vi "Build Edge Graph Legend.vi"() -> (3 "Edge Legend Graph":string)   [LabVIEW 2021, in "TAF Proj Document Type.lvlib" / "TAF Proj.lvclass"]
uses:
  <vilib>/Wovalab/AntiDoc/Document Type/Add-ons/LabVIEW TAF Project/TAF Proj/TAF Proj.lvclass
  <vilib>/Wovalab/AntiDoc/GraphBuilder/Renderer/Graphviz/Graphviz.lvclass
  C:/Program Files (x86)/National Instruments/LabVIEW 2021/vi.lib/Wovalab/AntiDoc/GraphBuilder/Renderer/Renderer.lvclass
  <vilib>/Wovalab/AntiDoc/GraphBuilder/Graph/Graph.lvclass
  <vilib>/Wovalab/AntiDoc/GraphBuilder/Shapes/Edge/Graphviz/Graphviz Edge Shape.lvclass
  <vilib>/Wovalab/AntiDoc/GraphBuilder/Shapes/Node/Graphviz/Graphviz Node Shape.lvclass
  <vilib>/Wovalab/AntiDoc/GraphBuilder/Shapes/Edge/Graphviz/Shape.ctl
  <vilib>/Wovalab/AntiDoc/GraphBuilder/Shapes/Edge/Graphviz/Colors.ctl
  <vilib>/Wovalab/AntiDoc/GraphBuilder/Shapes/Node/Graphviz/Colors.ctl
  <vilib>/Wovalab/AntiDoc/GraphBuilder/Shapes/Node/Graphviz/Shape.ctl
  <vilib>/Wovalab/AntiDoc/GraphBuilder/Renderer/Graphviz/Graph Direction.ctl
  <vilib>/Wovalab/AntiDoc/GraphBuilder/Edge/Edge.lvclass
  <vilib>/Wovalab/AntiDoc/GraphBuilder/Renderer/Graphviz/Specific Edge Shape Def.ctl
  <vilib>/Wovalab/AntiDoc/GraphBuilder/Node/Node.lvclass
  <vilib>/Wovalab/AntiDoc/GraphBuilder/Renderer/Graphviz/Specific Node Shape Def.ctl
  <vilib>/Wovalab/AntiDoc/Document Type/Add-ons/LabVIEW TAF Project/TAF Proj Document Type.lvlib
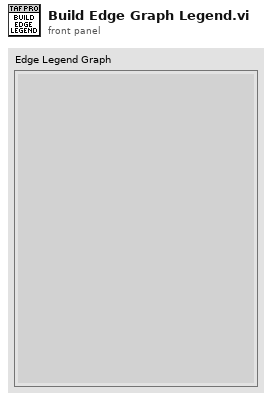
[diagram p1: front panel]
types:
  T1 = typedef "GraphBuilder.lvlib/Graphviz Edge Shape.lvclass/Shape.ctl" = enum16{"box", "lbox", "rbox", "obox", "olbox", "orbox", "crow", "lcrow", "rcrow", "diamond", "ldiamond", "rdiamond", "odiamond", "oldiamond", "ordiamond", "dot", "odot", "inv", "linv", "rinv", "oinv", "olinv", "orinv", "none", "normal", "lnormal", "rnormal", "onormal", "olnormal", "ornormal", "tee", "ltee", "rtee", "vee", "lvee", "rvee", "curve", "lcurve", "rcurve", "icurve", "licurve", "ricurve"}
  T2 = typedef "GraphBuilder.lvlib/Graphviz.lvclass/Specific Edge Shape Def.ctl" = cluster{"Source Node ID":string, "Target Node ID":string, "Caption":string, "Graphviz Edge Shape":refnum<class "Graphviz Edge Shape.lvclass">}
  T3 = typedef "GraphBuilder.lvlib/Graphviz.lvclass/Graph Direction.ctl" = enum16{"Top to Bottom", "Left To Right", "Bottom to Top", "Right to Left"}
  T4 = typedef "GraphBuilder.lvlib/Graphviz Node Shape.lvclass/Shape.ctl" = enum16{"box", "polygon", "ellipse", "oval", "circle", "point", "egg", "triangle", "plaintext", "plain", "diamond", "trapezium", "parallelogram", "house", "pentagon", "hexagon", "septagon", "octagon", "doublecircle", "doubleoctagon", "tripleoctagon", "invtriangle", "invtrapezium", "invhouse", "Mdiamond", "Msquare", "Mcircle", "rect", "rectangle", "square", "star", "none", "underline", "cylinder", "note", "tab", "folder", "box3D", "component", "promoter", "cds", "terminator", "utr", "primersite", "restrictionsite", "fivepoverhang", "threepoverhang", "noverhang", "assembly", "signature", "insulator", "ribosite", "rnastab", "proteasesite", "proteinstab", "rpromoter", "rarrow", "larrow", "lpromoter"}
  T5 = typedef "GraphBuilder.lvlib/Graphviz Node Shape.lvclass/Colors.ctl" = enum16{"aliceblue", "antiquewhite", "aqua", "aquamarine", "azure", "beige", "bisque", "black", "blanchedalmond", "blue", "blueviolet", "brown", "burlywood", "cadetblue", "chartreuse", "chocolate", "coral", "cornflowerblue", "cornsilk", "crimson", "cyan", "darkblue", "darkcyan", "darkgoldenrod", "darkgray", "darkgreen", "darkgrey", "darkkhaki", "darkmagenta", "darkolivegreen", "darkorange", "darkorchid", "darkred", "darksalmon", "darkseagreen", "darkslateblue", "darkslategray", "darkslategrey", "darkturquoise", "darkviolet", "deeppink", "deepskyblue", "dimgray", "dimgrey", "dodgerblue", "firebrick", "floralwhite", "forestgreen", "fuchsia", "gainsboro", "ghostwhite", "gold", "goldenrod", "gray", "green", "greenyellow", "grey", "honeydew", "hotpink", "indianred", "indigo", "ivory", "khaki", "lavender", "lavenderblush", "lawngreen", "lemonchiffon", "lightblue", "lightcoral", "lightcyan", "lightgoldenrodyellow", "lightgray", "lightgreen", "lightgrey", "lightpink", "lightsalmon", "lightseagreen", "lightskyblue", "lightslategray", "lightslategrey", "lightsteelblue", "lightyellow", "lime", "limegreen", "linen", "magenta", "maroon", "mediumaquamarine", "mediumblue", "mediumorchid", "mediumpurple", "mediumseagreen", "mediumslateblue", "mediumspringgreen", "mediumturquoise", "mediumvioletred", "midnightblue", "mintcream", "mistyrose", "moccasin", "navajowhite", "navy", "oldlace", "olive", "olivedrab", "orange", "orangered", "orchid", "palegoldenrod", "palegreen", "paleturquoise", "palevioletred", "papayawhip", "peachpuff", "peru", "pink", "plum", "powderblue", "purple", "red", "rosybrown", "royalblue", "saddlebrown", "salmon", "sandybrown", "seagreen", "seashell", "sienna", "silver", "skyblue", "slateblue", "slategray", "slategrey", "snow", "springgreen", "steelblue", "tan", "teal", "thistle", "tomato", "turquoise", "violet", "wheat", "white", "whitesmoke", "yellow", "yellowgreen"}
  T6 = typedef "GraphBuilder.lvlib/Graphviz Edge Shape.lvclass/Colors.ctl" = enum16{"aliceblue", "antiquewhite", "aqua", "aquamarine", "azure", "beige", "bisque", "black", "blanchedalmond", "blue", "blueviolet", "brown", "burlywood", "cadetblue", "chartreuse", "chocolate", "coral", "cornflowerblue", "cornsilk", "crimson", "cyan", "darkblue", "darkcyan", "darkgoldenrod", "darkgray", "darkgreen", "darkgrey", "darkkhaki", "darkmagenta", "darkolivegreen", "darkorange", "darkorchid", "darkred", "darksalmon", "darkseagreen", "darkslateblue", "darkslategray", "darkslategrey", "darkturquoise", "darkviolet", "deeppink", "deepskyblue", "dimgray", "dimgrey", "dodgerblue", "firebrick", "floralwhite", "forestgreen", "fuchsia", "gainsboro", "ghostwhite", "gold", "goldenrod", "gray", "green", "greenyellow", "grey", "honeydew", "hotpink", "indianred", "indigo", "ivory", "khaki", "lavender", "lavenderblush", "lawngreen", "lemonchiffon", "lightblue", "lightcoral", "lightcyan", "lightgoldenrodyellow", "lightgray", "lightgreen", "lightgrey", "lightpink", "lightsalmon", "lightseagreen", "lightskyblue", "lightslategray", "lightslategrey", "lightsteelblue", "lightyellow", "lime", "limegreen", "linen", "magenta", "maroon", "mediumaquamarine", "mediumblue", "mediumorchid", "mediumpurple", "mediumseagreen", "mediumslateblue", "mediumspringgreen", "mediumturquoise", "mediumvioletred", "midnightblue", "mintcream", "mistyrose", "moccasin", "navajowhite", "navy", "oldlace", "olive", "olivedrab", "orange", "orangered", "orchid", "palegoldenrod", "palegreen", "paleturquoise", "palevioletred", "papayawhip", "peachpuff", "peru", "pink", "plum", "powderblue", "purple", "red", "rosybrown", "royalblue", "saddlebrown", "salmon", "sandybrown", "seagreen", "seashell", "sienna", "silver", "skyblue", "slateblue", "slategray", "slategrey", "snow", "springgreen", "steelblue", "tan", "teal", "thistle", "tomato", "turquoise", "violet", "wheat", "white", "whitesmoke", "yellow", "yellowgreen"}
  T7 = typedef "GraphBuilder.lvlib/Graphviz.lvclass/Specific Node Shape Def.ctl" = cluster{"Node ID":string, "Graphviz Node Shape":refnum<class "Graphviz Node Shape.lvclass">}
  T8 = typedef "GraphBuilder.lvlib/Graphviz Edge Shape.lvclass/Style.ctl" = enum8{"filled", "invisible", "diagonals", "rounded", "dashed", "dotted", "solid", "bold"}
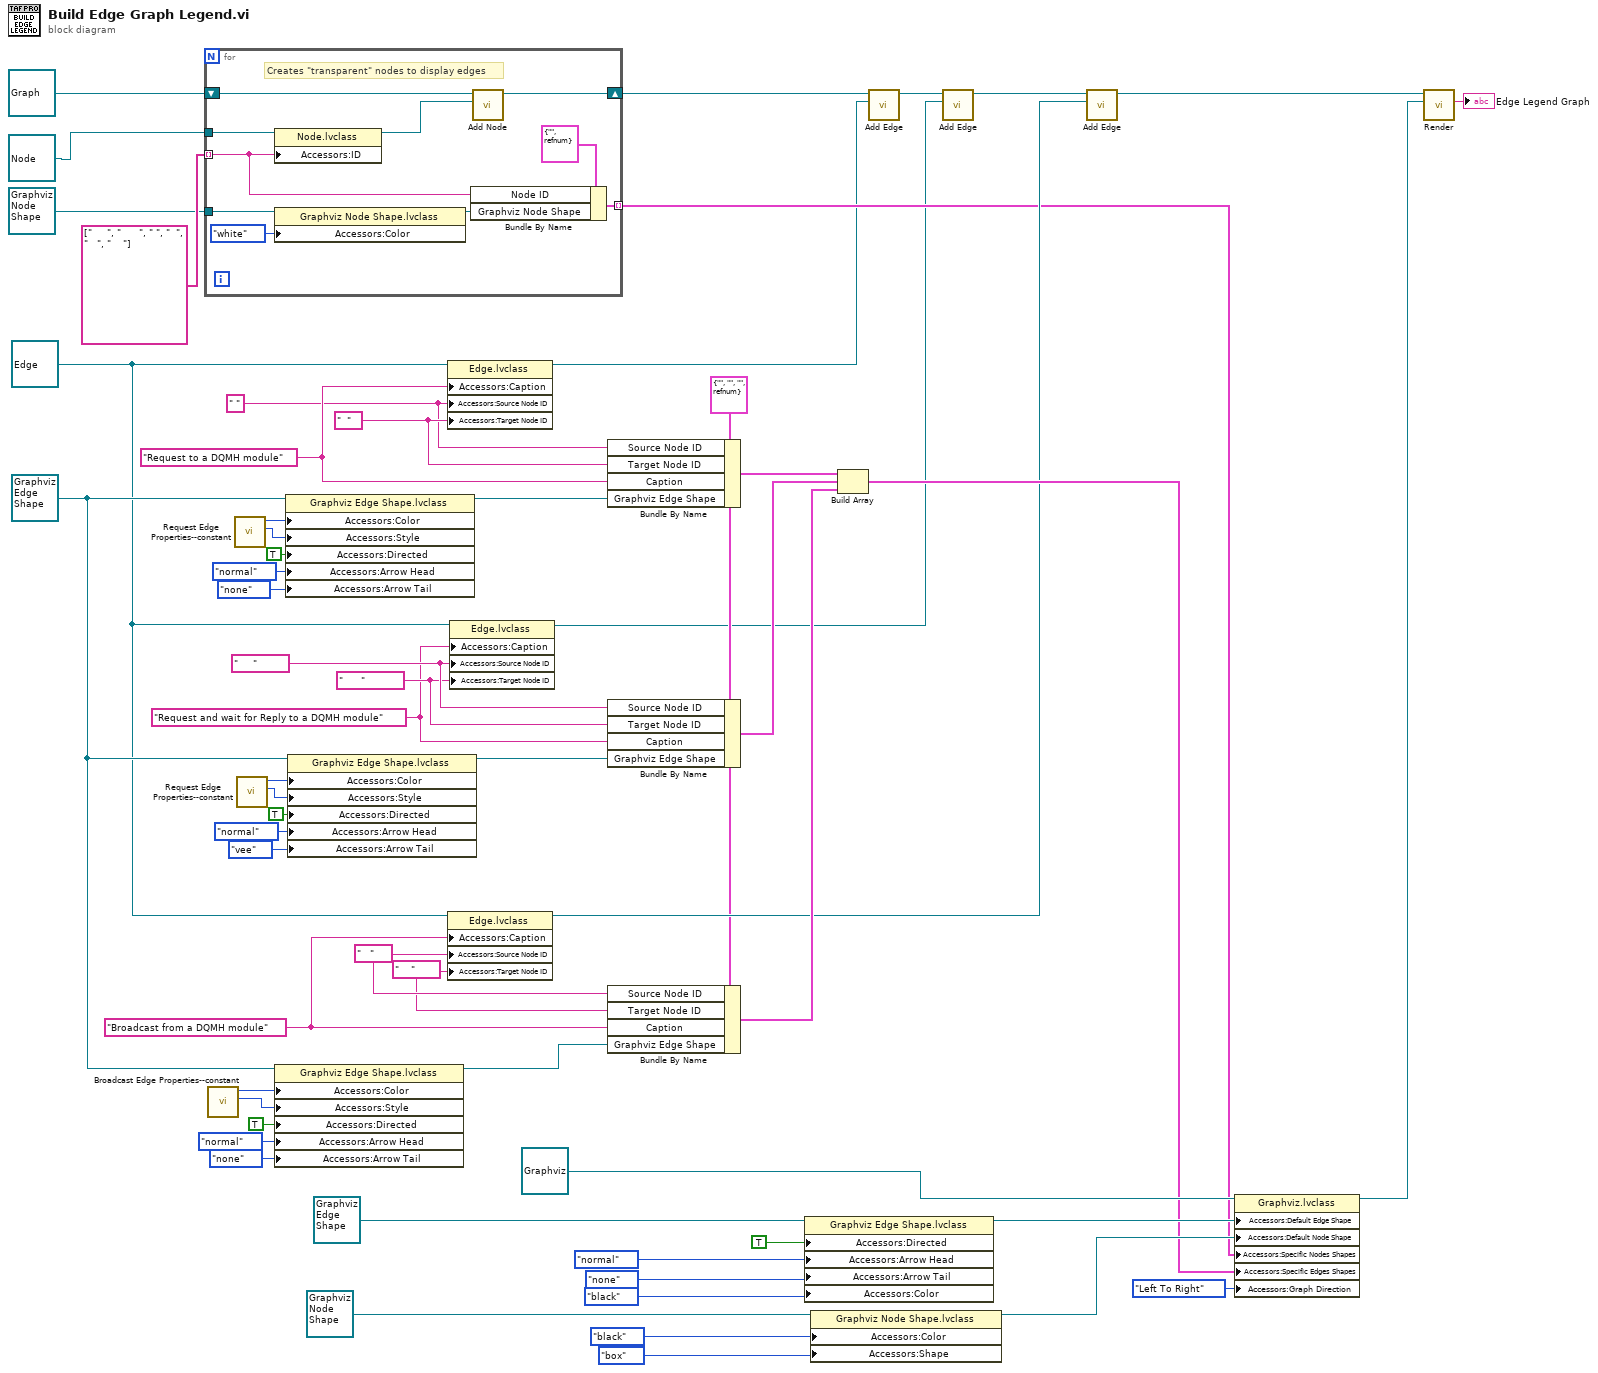
[diagram p0: block diagram]
diagram:
  w14 = "     "
  w13 = "      "
  w12 = "Request and wait for Reply to a DQMH module" ("Caption")
  w22 = " "
  w26 = "    "
  w27 = "   "
  w28 = "  "
  w38 = "Broadcast from a DQMH module" ("Caption")
  w5 = refnum<class "Graphviz Edge Shape.lvclass"> refnum ("Graphviz Edge Shape")
  w7 = T2 {"Source Node ID"="", "Target Node ID"="", "Caption"="", "Graphviz Edge Shape"=refnum} ("Specific Edge Shape")
  w32 = "Request to a DQMH module" ("Caption")
  w4 = refnum<class "Edge.lvclass"> refnum ("Edge")
  n1 = for {
    tunnel: string[] ["     ", "      ", " ", "  ", "   ", "    "] -> [w70] mode=indexing
    tunnel: [w66] -> w29 mode=indexing
    tunnel: refnum<class "Graphviz Node Shape.lvclass"> refnum ("GraphBuilder.lvlib:Graphviz Node Shape.lvclass") -> [w65]
    tunnel: refnum<class "Node.lvclass"> refnum ("GraphBuilder.lvlib:Node.lvclass") -> [w64]
    shift-right: [w62] -> w19
    shift-left: refnum<class "Graph.lvclass"> refnum ("GraphBuilder.lvlib:Graph.lvclass") -> [w63]
    # "Creates \"transparent\" nodes to display edges"
    n2 = property class="Node.lvclass"(reference=w64, "Accessors:ID"=w70) -> (reference out=w61:refnum<class "Node.lvclass">)  [unwired: 1 in, 1 out]
    n3 = property class="Graphviz Node Shape.lvclass"(reference=w65, "Accessors:Color"=Colors."white" ("Color")) -> (reference out=w69:refnum<class "Graphviz Node Shape.lvclass">)  [unwired: 1 in, 1 out]
    n4 = Bundle By Name(cluster=T7 {"Node ID"="", "Graphviz Node Shape"=refnum} ("Specific Node Shape"), "Node ID"=w70, "Graphviz Node Shape"=w69) -> (w66:T7)
    n5 = call-dynamic "Add Node.vi"("Node"=w61, "Graph in"=w63) -> ("Graph out"=w62:refnum<class "Graph.lvclass">)  [unwired: 8 in, 1 out]
  }
  n6 = call <vilib>:"Broadcast Edge Properties--constant.vi"() -> ("Style"=w35:T8, "Edge Color"=w36:T6)  [unwired: 10 in]
  n7 = call <vilib>:"Request Edge Properties--constant.vi"() -> ("Style"=w45:T8, "Edge Color"=w46:T6)  [unwired: 10 in]
  n8 = call <vilib>:"Request Edge Properties--constant.vi"() -> ("Style"=w10:T8, "Edge Color"=w9:T6)  [unwired: 10 in]
  n9 = property class="Graphviz Edge Shape.lvclass"(reference=w5, "Accessors:Color"=w36, "Accessors:Style"=w35, "Accessors:Directed"=TRUE ("Directed"), "Accessors:Arrow Head"=Shape."normal" ("Arrow Head"), "Accessors:Arrow Tail"=Shape."none" ("Arrow Tail")) -> (reference out=w39:refnum<class "Graphviz Edge Shape.lvclass">)  [unwired: 1 in, 1 out]
  n10 = property class="Graphviz Edge Shape.lvclass"(reference=w5, "Accessors:Color"=w46, "Accessors:Style"=w45, "Accessors:Directed"=TRUE ("Directed"), "Accessors:Arrow Head"=Shape."normal" ("Arrow Head"), "Accessors:Arrow Tail"=Shape."none" ("Arrow Tail")) -> (reference out=w47:refnum<class "Graphviz Edge Shape.lvclass">)  [unwired: 1 in, 1 out]
  n11 = property class="Graphviz Edge Shape.lvclass"(reference=w5, "Accessors:Color"=w9, "Accessors:Style"=w10, "Accessors:Directed"=TRUE ("Directed"), "Accessors:Arrow Head"=Shape."normal" ("Arrow Head"), "Accessors:Arrow Tail"=Shape."vee" ("Arrow Tail")) -> (reference out=w8:refnum<class "Graphviz Edge Shape.lvclass">)  [unwired: 1 in, 1 out]
  n12 = property class="Edge.lvclass"(reference=w4, "Accessors:Caption"=w32, "Accessors:Source Node ID"=w22, "Accessors:Target Node ID"=w28) -> (reference out=w23:refnum<class "Edge.lvclass">)  [unwired: 1 in, 1 out]
  n13 = property class="Edge.lvclass"(reference=w4, "Accessors:Caption"=w38, "Accessors:Source Node ID"=w27, "Accessors:Target Node ID"=w26) -> (reference out=w34:refnum<class "Edge.lvclass">)  [unwired: 1 in, 1 out]
  n14 = property class="Edge.lvclass"(reference=w4, "Accessors:Caption"=w12, "Accessors:Source Node ID"=w14, "Accessors:Target Node ID"=w13) -> (reference out=w1:refnum<class "Edge.lvclass">)  [unwired: 1 in, 1 out]
  n15 = Bundle By Name(cluster=w7, "Source Node ID"=w22, "Target Node ID"=w28, "Caption"=w32, "Graphviz Edge Shape"=w47) -> (w43:T2)
  n16 = Bundle By Name(cluster=w7, "Source Node ID"=w14, "Target Node ID"=w13, "Caption"=w12, "Graphviz Edge Shape"=w8) -> (w6:T2)
  n17 = Bundle By Name(cluster=w7, "Source Node ID"=w27, "Target Node ID"=w26, "Caption"=w38, "Graphviz Edge Shape"=w39) -> (w37:T2)
  n18 = property class="Graphviz Edge Shape.lvclass"(reference=refnum<class "Graphviz Edge Shape.lvclass"> refnum ("GraphBuilder.lvlib:Graphviz Edge Shape.lvclass"), "Accessors:Directed"=TRUE ("Directed"), "Accessors:Arrow Head"=Shape."normal" ("Arrow Head"), "Accessors:Arrow Tail"=Shape."none" ("Arrow Tail"), "Accessors:Color"=Colors."black" ("Color")) -> (reference out=w58:refnum<class "Graphviz Edge Shape.lvclass">)  [unwired: 1 in, 1 out]
  n19 = property class="Graphviz Node Shape.lvclass"(reference=refnum<class "Graphviz Node Shape.lvclass"> refnum ("GraphBuilder.lvlib:Graphviz Node Shape.lvclass"), "Accessors:Color"=Colors."black" ("Color"), "Accessors:Shape"=Shape."box" ("Shape")) -> (reference out=w59:refnum<class "Graphviz Node Shape.lvclass">)  [unwired: 1 in, 1 out]
  n20 = Build Array(w43, w6, w37) -> (w42:T2[])
  n21 = call-dynamic "Add Edge.vi"("Edge"=w23, "Graph in"=w19) -> ("Graph out"=w3:refnum<class "Graph.lvclass">)  [unwired: 8 in, 1 out]
  n22 = call-dynamic "Add Edge.vi"("Edge"=w1, "Graph in"=w3) -> ("Graph out"=w2:refnum<class "Graph.lvclass">)  [unwired: 8 in, 1 out]
  n23 = call-dynamic "Add Edge.vi"("Edge"=w34, "Graph in"=w2) -> ("Graph out"=w41:refnum<class "Graph.lvclass">)  [unwired: 8 in, 1 out]
  n24 = property class="Graphviz.lvclass"(reference=refnum<class "Graphviz.lvclass"> refnum ("GraphBuilder.lvlib:Graphviz.lvclass"), "Accessors:Default Edge Shape"=w58, "Accessors:Default Node Shape"=w59, "Accessors:Specific Nodes Shapes"=w29, "Accessors:Specific Edges Shapes"=w42, "Accessors:Graph Direction"=Graph_Direction."Left To Right" ("Graph Direction")) -> (reference out=w60:refnum<class "Graphviz.lvclass">)  [unwired: 1 in, 1 out]
  n25 = call-dynamic "Render.vi"("Renderer"=w60, "Graph in"=w41) -> ("Rendered Stream"=→"Edge Legend Graph":string)  [unwired: 7 in, 2 out]
